vi "获取标签第一个属性.vi"(6 "error in (no error)":errorcluster caption="错误输入（无错误）", 8 "offset (0)":i32 caption="偏移量(0)", 11 "XML String In":string caption="XML字符串输入") -> (0 "offset past match":i32 caption="匹配后偏移量", 1 "after  tag":string caption="标识符之后", 2 "tag":string caption="标识符", 3 "node name":string caption="节点名称", 4 "error out":errorcluster caption="错误输出", 5 "attribute value":string caption="属性值", 7 "attribute name":string caption="属性名")   [LabVIEW 2017]
uses:
  <vilib>/Utility/error.llb/whitespace.ctl
  <vilib>/regexp/Match Regular Expression.xnode
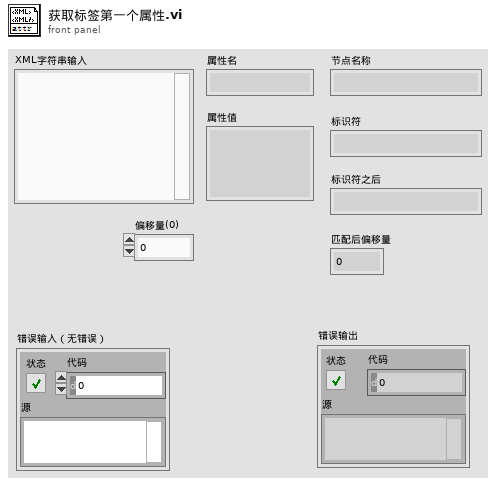
[diagram p1: front panel]
types:
  T1 = typedef "whitespace.ctl" = u16
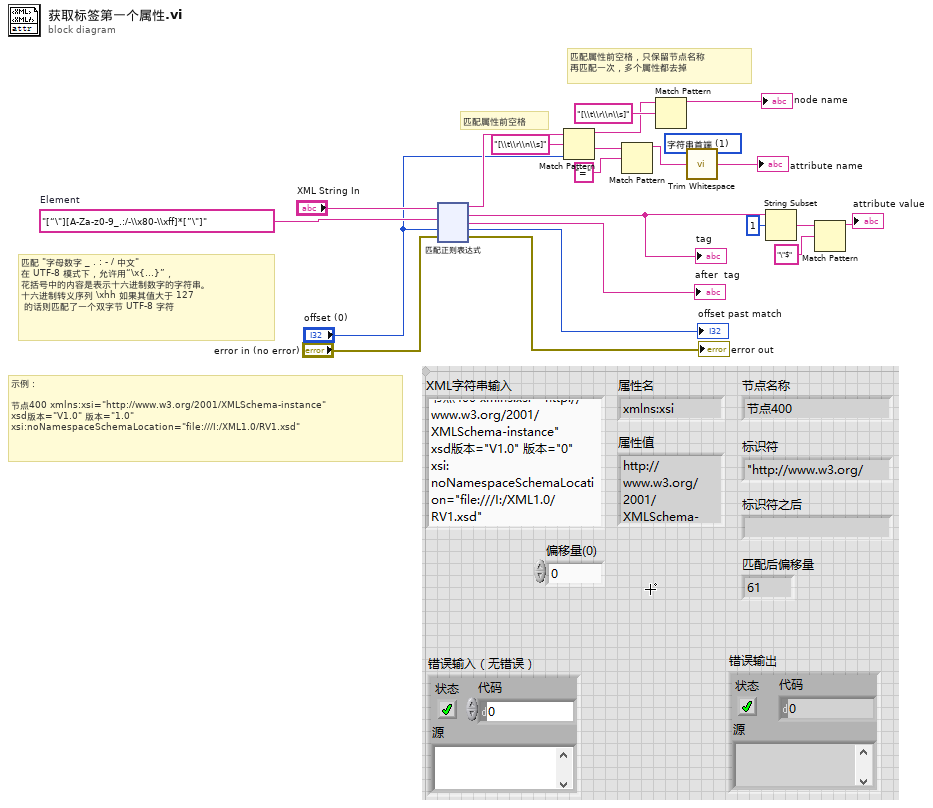
[diagram p0: block diagram]
diagram:
  w1 = T1 1 items=["两端", "字符串首端", "字符串末端"] ("location (both)")
  w20 = "[“\"][A-Za-z0-9_.:/-\\x80-\\xff]*[”\"]"  # Element
  # "示例：\n\n节点400 xmlns:xsi=\"http://www.w3.org/2001/XMLSchema-instance\" \nxsd版本=\"V1.0\" 版本=\"1.0\" \nxsi:noNamespaceSchemaLocation=\"file:///I:/XML1.0/RV1.xsd\""
  # "匹配属性前空格，只保留节点名称\n再匹配一次，多个属性都去掉"
  # "匹配属性前空格"
  # "匹配 \"字母数字 _ . : - / 中文\"\n在 UTF-8 模式下，允许用“\\x{...}”，\n花括号中的内容是表示十六进制数字的字符串。\n十六进制转义序列 \\xhh 如果其值大于 127\n 的话则匹配了一个双字节 UTF-8 字符"
  n1 = xnode "匹配正则表达式"("输入字符串"="XML String In", "正则表达式"=w20, "偏移量(0)"="offset (0)", "错误输入"="error in (no error)") -> ("匹配之前"=w13:string, "所有匹配"=w19:string, "匹配之后"=→"after  tag":string, "匹配后偏移量"=→"offset past match":i32, "错误输出"=→"error out":errorcluster)  [unwired: 2 in]
  "tag" <- w19
  n2 = Match Pattern(string=w13, regular expression="[\\t\\r\\n\\s]" ("正则表达式"), offset (0)="offset (0)") -> (before substring=w5:string, after substring=w12:string)  [unwired: 2 out]
  n3 = Match Pattern(string=w12, regular expression="=" ("正则表达式")) -> (before substring=w3:string)  [unwired: 1 in, 3 out]
  n4 = Match Pattern(string=w5, regular expression="[\\t\\r\\n\\s]" ("正则表达式")) -> (before substring=→"node name":string)  [unwired: 1 in, 3 out]
  n5 = call <vilib>:"Trim Whitespace.vi"("string"=w3, "location (both)"=w1) -> ("trimmed string"=→"attribute name":string)
  n6 = String Subset(string=w19, offset (0)=1) -> (substring=w16:string)  [unwired: 1 in]
  n7 = Match Pattern(string=w16, regular expression="\"$" ("正则表达式")) -> (before substring=→"attribute value":string)  [unwired: 1 in, 3 out]
